vi "Compass.vi"() -> (0 "Error Out":errorcluster)   [LabVIEW 2017]
uses:
  <vilib>/Platform/TimedLoop/XDataNode/timing_clust.ctl
  <vilib>/Platform/TimedLoop/XDataNode/nitl_modes.ctl
  <vilib>/Platform/TimedLoop/XDataNode/wakeup.ctl
  <vilib>/myRIO/Instrument Drivers/Onboard IO/I2C/typedefs/I2C User Configuration.ctl
  <vilib>/myRIO/Instrument Drivers/Onboard IO/I2C/typedefs/I2C Transfer Rate.ctl
  <vilib>/myRIO/Instrument Drivers/Onboard IO/I2C/typedefs/I2C Reference.ctl
  <vilib>/myRIO/Common/Instrument Driver Framework/Utilities/typedefs/myRIO Generic Hardware Reference.ctl
  <vilib>/myRIO/Common/Instrument Driver Framework/Utilities/typedefs/Hardware Version Enum.ctl
  <vilib>/myRIO/Common/Instrument Driver Framework/Utilities/typedefs/myRIO v1.0 Reference.ctl
  <vilib>/myRIO/Common/Instrument Driver Framework/Utilities/typedefs/Generic FPGA Reference.ctl
  <vilib>/myRIO/Common/Instrument Driver Framework/myRIO v1.0/I2C/typedefs/I2C Channels Enum.ctl
  <vilib>/myRIO/Instrument Drivers/Onboard IO/I2C/typedefs/I2C Configuration.ctl
  <vilib>/userdefined/High Color/nirio_resource_hc.ctl
  <vilib>/myRIO/Instrument Drivers/Onboard IO/DIO/typedefs/DIO Reference.ctl
  <vilib>/myRIO/Common/Instrument Driver Framework/myRIO v1.0/DIO/typedefs/DIO Channels List.ctl
  <vilib>/myRIO/Common/Instrument Driver Framework/myRIO v1.0/DIO/typedefs/DIO Channels Enum.ctl
  <vilib>/myRIO/Common/Instrument Driver Framework/Utilities/vis/Is FPGA Ref Available.vi
  <vilib>/myRIO/Common/Instrument Driver Framework/myRIO v1.0/I2C/vis/myRIO v1.1 Open I2C.vi
  <vilib>/myRIO/Instrument Drivers/Onboard IO/I2C/vis/Configure.vi
  <vilib>/myRIO/Instrument Drivers/Onboard IO/I2C/vis/Write.vi
  <vilib>/myRIO/Common/Instrument Driver Framework/myRIO v1.0/DIO/vis/myRIO v1.1 Open DIO.vi
  <vilib>/myRIO/Instrument Drivers/Onboard IO/DIO/vis/Read.vi
  <vilib>/myRIO/Common/Instrument Driver Framework/Utilities/vis/Validate Channels.vi
  <vilib>/myRIO/Common/Instrument Driver Framework/myRIO v1.0/I2C/vis/myRIO v1.0 Reserve I2C.vi
  <vilib>/myRIO/Common/Instrument Driver Framework/myRIO v1.0/DIO/vis/myRIO v1.0 Reserve DIO.vi
  <vilib>/myRIO/Instrument Drivers/Onboard IO/I2C/vis/Write Read.vi
  <vilib>/myRIO/Common/Instrument Driver Framework/myRIO v1.0/I2C/vis/myRIO v1.0 Build MUX Configuration I2C.vi
  <vilib>/myRIO/Common/Instrument Driver Framework/myRIO v1.0/Resource Manager/vis/myRIO v1.0 Reserve Channel List.vi
  <vilib>/myRIO/Common/Instrument Driver Framework/myRIO v1.0/DIO/vis/myRIO v1.0 Build MUX Configuration DIO.vi
  <vilib>/myRIO/Common/Instrument Driver Framework/myRIO v1.0/Resource Manager/vis/myRIO v1.0 Create Configuration List.vi
  <vilib>/myRIO/Common/Instrument Driver Framework/myRIO v1.0/Resource Manager/vis/myRIO v1.0 Reserve Channel.vi
  <vilib>/myRIO/Common/Instrument Driver Framework/myRIO v1.0/Resource Manager/vis/myRIO v1.0 Unreserve Channel.vi
  <vilib>/myRIO/Common/Instrument Driver Framework/myRIO v1.0/Resource Manager/vis/myRIO v1.0 Build Mutex Name.vi
  <vilib>/Utility/VariantDataType/GetNumericInfo.vi
  <vilib>/Utility/error.llb/Error Cluster From Error Code.vi
  <vilib>/myRIO/Common/Instrument Driver Framework/myRIO v1.0/myRIO v1.1 Open.vi
  <vilib>/myRIO/Common/Instrument Driver Framework/Utilities/vis/IO Manager.vi
  <vilib>/myRIO/Common/Instrument Driver Framework/Utilities/vis/Configuration Manager.vi
  <vilib>/myRIO/Common/Instrument Driver Framework/myRIO v1.0/Resource Manager/vis/myRIO v1.0 Configure IO.vi
  <vilib>/myRIO/Common/Instrument Driver Framework/myRIO v1.0/myRIO v1.0 Close.vi
  <vilib>/myRIO/Common/Instrument Driver Framework/myRIO v1.0/I2C/vis/myRIO v1.0 Configure I2C.vi
  <vilib>/myRIO/Common/Instrument Driver Framework/myRIO v1.0/I2C/vis/myRIO v1.0 Write I2C.vi
  <vilib>/myRIO/Common/Instrument Driver Framework/myRIO v1.0/DIO/vis/myRIO v1.0 Read DIO.vi
  <vilib>/myRIO/Instrument Drivers/Onboard IO/I2C/vis/Smart Open.vi
  <vilib>/myRIO/Common/Instrument Driver Framework/myRIO v1.0/I2C/vis/myRIO v1.0 Read I2C.vi
  <vilib>/Platform/TimedLoop/XDataNode/XDataNode.xnode
  <vilib>/myRIO/Express VI/Onboard IO/I2C/I2C Express VI.xnode
  <vilib>/myRIO/Instrument Drivers/Onboard IO/I2C/vis/myRIO I2C Open.xnode
  <vilib>/myRIO/Express VI/Onboard IO/DI/DI Express VI.xnode
  <vilib>/myRIO/Instrument Drivers/Onboard IO/DIO/vis/myRIO DIO Open.xnode
  <vilib>/Platform/TimedLoop/XDataNode/XDNodeRunTimeDep.lvlib
  <vilib>/myRIO/Instrument Drivers/Onboard IO/I2C/I2C.lvlib
  <vilib>/myRIO/Instrument Drivers/Onboard IO/DIO/DIO.lvlib
panel:
  out "Angle (deg) without declination added":dbl
  out "Angle + 90 (deg)":dbl
  out "Angle (deg)":dbl
  out "atan2(y,x)":dbl
  out "cali_Y":dbl
  out "cali_X":dbl
  out "avg(Y)":dbl
  out "avg(X)":dbl
  out "max(Y)":i16
  out "min(Y)":i16
  out "min(X)":i16
  out "max(X)":i16
  out "Magnetic field [LSb]":cluster{i16, i16, i16}(graph) caption="Waveform Chart"
  out "Z":i16
  out "Y":i16
  out "X":i16
  out "DATA":u8[](array[numeric]) format="%02x"
  # "Compass demo"
  # "DATA_X_H"
  # "DATA_X_L"
  # "DATA_Z_H"
  # "DATA_Z_L"
  # "DATA_Y_H"
  # "DATA_Y_L"
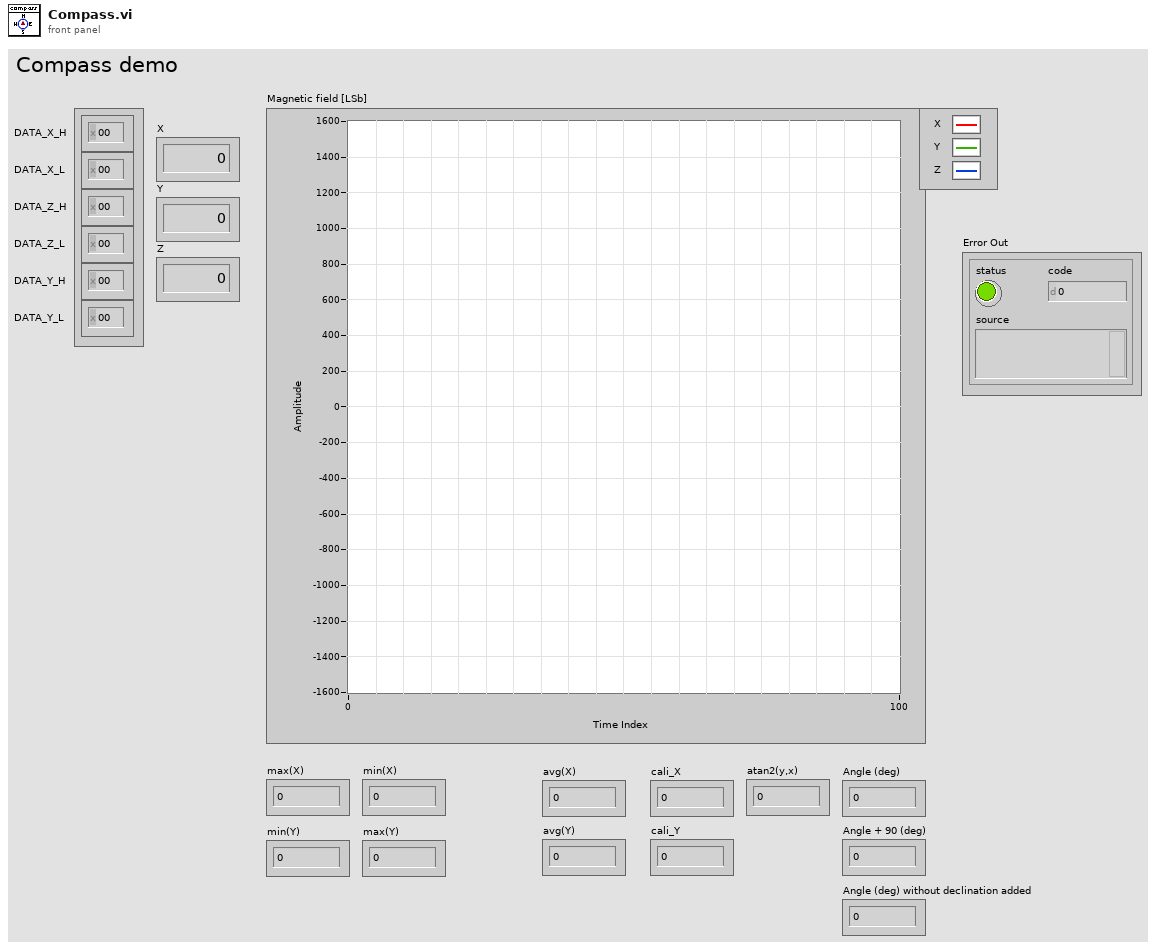
[diagram p1: front panel]
types:
  T1 = typedef "XDNodeRunTimeDep.lvlib/timing_clust.ctl" = cluster{"Expected End [f-1]":u64, "Actual End [f-1]":u64, "Finished Late? [f-1]":bool, "Expected End [i-1]":u64, "Actual End [i-1]":u64, "Finished Late? [i-1]":bool, "Expected Start [i]":u64, "Actual Start [i]":u64, "Expected Start [f]":u64, "Actual Start [f]":u64, "Source Name":string, "Structure Name":string, "Period":i64, "Deadline":i64, "Offset":i64, "Start":i64, "Priority":i32, "Timeout":i32, "Mode":T2, "Wakeup Reason":T3, "Error":errorcluster, "Source Type":string, "Secondary Source Type":string, "Global End Time":u64, "Global Start Time":u64, "Frame Duration":u64, "Iteration Duration":u64, "Assigned CPU":i32, "I/O Scan Engine Mode":u32}
  T2 = typedef "XDNodeRunTimeDep.lvlib/nitl_modes.ctl" = enum32{"No Change", "Process missed periods, maintain original phase", "Discard missed periods, maintain original phase", "Process missed periods, ignore original phase", "Discard missed periods, ignore original phase"}
  T3 = typedef "XDNodeRunTimeDep.lvlib/wakeup.ctl" = enum32{"Normal", "Aborted", "Asynchronous wakeup", "Timing source error", "Timed loop error", "Timeout"}
  T4 = typedef "DIO.lvlib/DIO Reference.ctl" = cluster{"myRIO Reference":T5, "DIO Channels List":T9}
  T5 = typedef "myRIO Generic Hardware Reference.ctl" = cluster{"myRIO Model":T6, "myRIO Hardware Reference":T7}
  T6 = typedef "Hardware Version Enum.ctl" = enum16{"Unknown", "myRIO-1900", "myRIO-1950", "roboRIO", "NI ELVIS RIO CM"}
  T7 = typedef "myRIO v1.0 Reference.ctl" = cluster{"Generic FPGA Reference":T8, "Allow multiple opens":bool}
  T8 = typedef "Generic FPGA Reference.ctl" = refnum<k20>
  T9 = typedef "DIO Channels List.ctl" = T10[]
  T10 = typedef "DIO Channels Enum.ctl" = enum16{"Not Connected", "C/DIO0", "C/DIO1", "C/DIO2", "C/DIO3", "C/DIO4", "C/DIO5", "C/DIO6", "C/DIO7", "A/DIO0", "A/DIO1", "A/DIO2", "A/DIO3", "A/DIO4", "A/DIO5", "A/DIO6", "A/DIO7", "A/DIO8", "A/DIO9", "A/DIO10", "A/DIO11", "A/DIO12", "A/DIO13", "A/DIO14", "A/DIO15", "B/DIO0", "B/DIO1", "B/DIO2", "B/DIO3", "B/DIO4", "B/DIO5", "B/DIO6", "B/DIO7", "B/DIO8", "B/DIO9", "B/DIO10", "B/DIO11", "B/DIO12", "B/DIO13", "B/DIO14", "B/DIO15", "LED0", "LED1", "LED2", "LED3", "Button0", "DIO/DIO0", "DIO/DIO1", "DIO/DIO2", "DIO/DIO3", "DIO/DIO4", "DIO/DIO5", "DIO/DIO6", "DIO/DIO7", "DIO/DIO8", "DIO/DIO9", "SPI/CS0", "SPI/CS1", "SPI/CS2", "SPI/CS3", "LED RADIO (Green)", "LED RADIO (Red)", "LED COMM (Green)", "LED COMM (Red)", "LED MODE (Green)", "LED MODE (Red)"}
  T11 = typedef "nirio_resource_hc.ctl" = tag
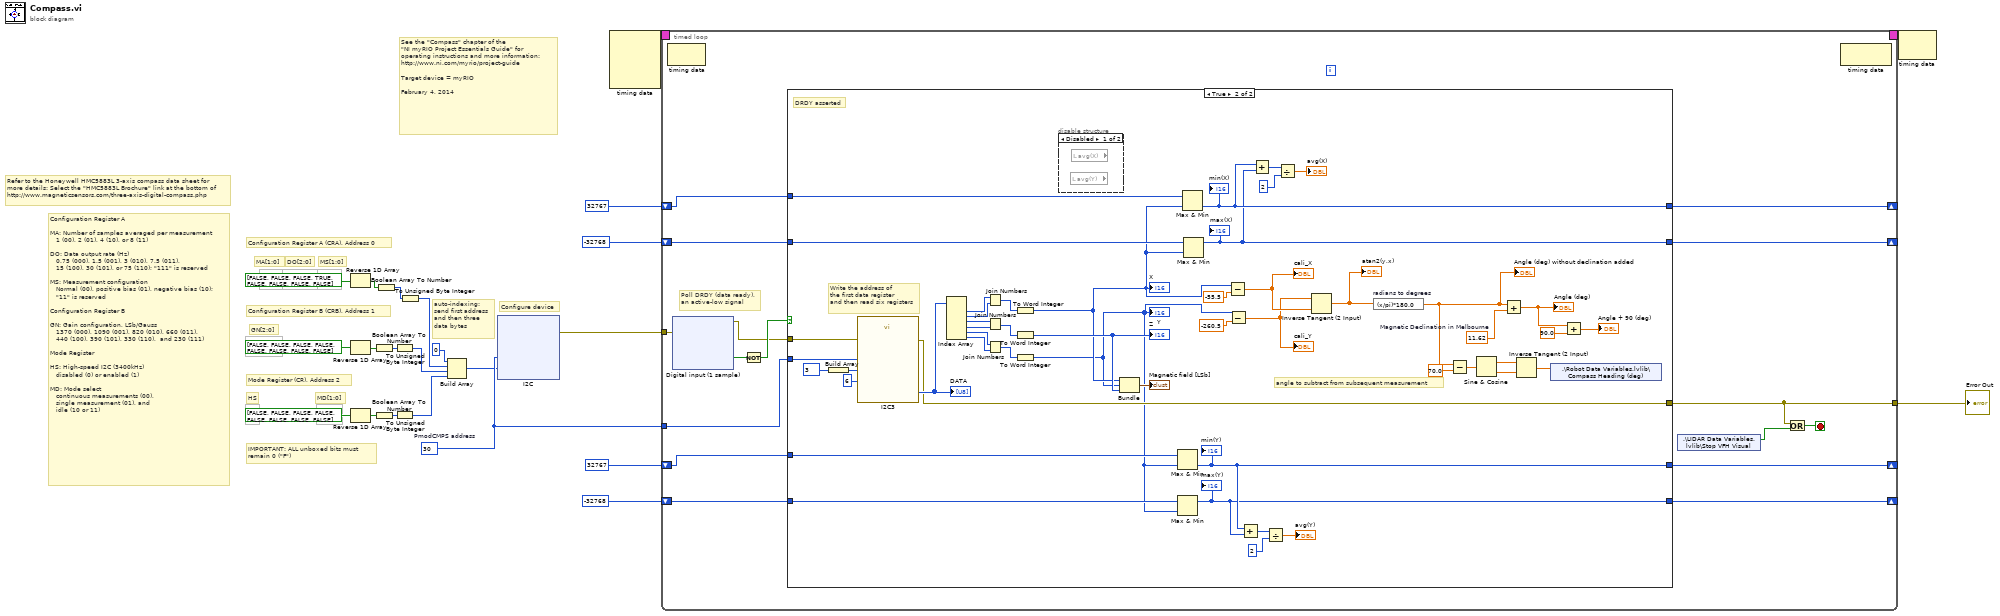
[diagram p0: block diagram]
diagram:
  w22 = u8 30  # PmodCMPS address
  # "See the \"Compass\" chapter of the\n\"NI myRIO Project Essentials Guide\" for\noperating instructions and more information: \nhttp://www.ni.com/myrio/project-guide\n\nTarget device = myRIO\n\nFebruary 4, 2014"
  # "Refer to the Honeywell HMC5883L 3-axis compass data sheet for \nmore details: Select the \"HMC5883L Brochure\" link at the bottom of\nhttp://www.magneticsensors.com/three-axis-digital-compass.php"
  # "auto-indexing:\nsend first address\nand then three\ndata bytes"
  # "Configuration Register A\n\nMA: Number of samples averaged per measurement\n   1 (00), 2 (01), 4 (10), or 8 (11)\n\nDO: Data output rate (Hz)\n   0.75 (000), 1.5 (001), 3 (010), 7.5 (011),\n   15 (100), 30 (101), or 75 (110); \"111\" is reserved\n\nMS: Measurement configuration\n   Normal (00), positive bias (01), negative bias (10);\n   \"11\" is reserved\n\nConfiguration Register B\n\nGN: Gain configuration, LSb/Gauss\n   1370 (000), 1090 (001), 820 (010), 660 (011),\n   440 (100), 390 (101), 330 (110),  and 230 (111)\n\nMode Register\n\nHS: High-speed I2C (3400kHz)\n   disabled (0) or enabled (1)\n\nMD: Mode select\n   continuous measurements (00),\n   single measurement (01), and\n   idle (10 or 11)"
  # "IMPORTANT: ALL unboxed bits must\nremain 0 (\"F\")"
  # "Configure device"
  # "MD[1:0]"
  # "Mode Register (CR), Address 2"
  # "HS"
  # "Configuration Register B (CRB), Address 1"
  # "GN[2:0]"
  # "Configuration Register A (CRA), Address 0"
  # "MS[1:0]"
  # "DO[2:0]"
  # "MA[1:0]"
  n1 = Reverse 1D Array(array=bool[] [FALSE, FALSE, FALSE, TRUE, FALSE, FALSE, FALSE, FALSE]) -> (reversed array=w17:bool[])
  n2 = Reverse 1D Array(array=bool[] [FALSE, FALSE, FALSE, FALSE, FALSE, FALSE, FALSE, FALSE]) -> (reversed array=w16:bool[])
  n3 = Reverse 1D Array(array=bool[] [FALSE, FALSE, FALSE, FALSE, FALSE, FALSE, FALSE, FALSE]) -> (reversed array=w14:bool[])
  n4 = Boolean Array To Number(Boolean array=w16) -> (number=w10:u32)
  n5 = Boolean Array To Number(Boolean array=w14) -> (number=w9:u32)
  n6 = Boolean Array To Number(Boolean array=w17) -> (number=w11:u32)
  n7 = To Unsigned Byte Integer(number=w10) -> (unsigned 8bit integer=w7:u8)
  n8 = To Unsigned Byte Integer(number=w9) -> (unsigned 8bit integer=w6:u8)
  n9 = To Unsigned Byte Integer(number=w11) -> (unsigned 8bit integer=w8:u8)
  n10 = Build Array "Build Array"(u8 0 ("address"), w8, w7, w6) -> (w21:u8[])
  n11 = xnode "I2C"("Slave Address (7-bit)"=w22, "Bytes to Write"=w21) -> ("error out"=w23:errorcluster)  [unwired: 1 in]
  n12 = node-c288() -> (w20:T1)  [unwired: 4 in]
  n13 = timed-loop {
    tunnel: [w33] -> w1
    tunnel: w23 -> [w37]
    tunnel: w22 -> [w38]
    timing: w20 -> [_]
    timing-out: [_] -> w19
    shift-right: [w32] -> _
    shift-left: i16 -32768 -> [w31]
    shift-right: [w30] -> _
    shift-left: i16 32767 -> [w29]
    shift-right: [w27] -> _
    shift-left: i16 32767 -> [w26]
    shift-right: [w28] -> _
    shift-left: i16 -32768 -> [w25]
    stop <- w39 stop-if-true
    # "Poll DRDY (data ready),\nan active-low signal"
    n14 = node-c288() -> ()  [unwired: 1 in, 1 out]
    n15 = xnode "Digital input (1 sample)"("error in (no error)"=w37) -> ("A/DIO7 (Pin 25)"=w36:bool, "error out"=w34:errorcluster)
    n16 = Not(x=w36) -> (.not. x?=w35:bool)
    n17 = case shown="True" w35 {
      tunnel: w38 -> [_ w130]
      tunnel: w34 -> [w81 w119]
      tunnel: [w81 w115] -> w33
      tunnel: [w80 w106] -> w32
      tunnel: w31 -> [w80 w113]
      tunnel: [w79 w107] -> w30
      tunnel: w29 -> [w79 w111]
      tunnel: [w77 w100] -> w28
      tunnel: [w78 w101] -> w27
      tunnel: w26 -> [w78 w110]
      tunnel: w25 -> [w77 w109]
      frame False {
        # "DRDY deasserted"
      }
      frame True {
        w93 = 11.62  # Magnetic Declination in Melbourne
        # "angle to subtract from subsequent measurement"
        # "DRDY asserted"
        # "Write the address of\nthe first data register\nand then read six registers"
        n18 = Build Array(u8 3) -> (w116:u8[])
        n19 = call "I2C3"("Slave Address (7-bit)"=w130, "Bytes to Write"=w116, "Byte Count"=u32 6, "error in (no error)"=w119) -> ("Bytes Read"=w120:u8[], "error out"=w115:errorcluster)  [unwired: 22 in]
        "DATA" <- w120
        n20 = Index Array "Index Array"(array=w120) -> (element #1=w129:u8, element #2=w128:u8, element #3=w126:u8, element #4=w125:u8, element #5=w124:u8, element #6=w123:u8)  [unwired: 6 in]
        n21 = Join Numbers(hi=w129, lo=w128) -> ((hi.lo)=w127:u16)
        n22 = Join Numbers(hi=w126, lo=w125) -> ((hi.lo)=w122:u16)
        n23 = Join Numbers(hi=w124, lo=w123) -> ((hi.lo)=w121:u16)
        n24 = To Word Integer(number=w127) -> (16bit integer=w98:i16)
        "X" <- w98
        n25 = To Word Integer(number=w122) -> (16bit integer=w112:i16)
        "Z" <- w112
        n26 = To Word Integer(number=w121) -> (16bit integer=w97:i16)
        "Y" <- w97
        n27 = disable-structure shown="Disabled" {
          frame Disabled {
            n28 = local read "avg(Y)"() -> ()  [unwired: 1 out]
            n29 = local read "avg(X)"() -> ()  [unwired: 1 out]
          }
          frame Enabled {
          }
        }
        n30 = Bundle(w98, w97, w112) -> (→"Magnetic field [LSb]":cluster{i16, i16, i16})  [unwired: 1 in]
        n31 = Max & Min(x=w110, y=w97) -> (min(x,y)=w101:i16)  [unwired: 1 out]
        "min(Y)" <- w101
        n32 = Max & Min(x=w109, y=w97) -> (max(x,y)=w100:i16)  [unwired: 1 out]
        "max(Y)" <- w100
        n33 = Max & Min(x=w111, y=w98) -> (min(x,y)=w107:i16)  [unwired: 1 out]
        "min(X)" <- w107
        n34 = Max & Min(x=w113, y=w98) -> (max(x,y)=w106:i16)  [unwired: 1 out]
        "max(X)" <- w106
        n35 = Subtract(x=w98, y=-55.5 ("Magnetic Declination in Melbourne")) -> (x-y=w95:dbl)
        "cali_X" <- w95
        n36 = Subtract(x=w97, y=-260.5 ("Magnetic Declination in Melbourne")) -> (x-y=w94:dbl)
        "cali_Y" <- w94
        n37 = Add(x=w101, y=w100) -> (x+y=w103:i16)
        n38 = Add(x=w107, y=w106) -> (x+y=w108:i16)
        n39 = Divide(x=w103, y=i16 2) -> (x/y=→"avg(Y)":dbl)
        n40 = Divide(x=w108, y=i16 2) -> (x/y=→"avg(X)":dbl)
        n41 = Inverse Tangent (2 Input)(1:w95, 2:w94) -> (0:w96:dbl)
        "atan2(y,x)" <- w96
        n42 = expression code="(x/pi)*180.0" "radians to degrees"(w96) -> (w87:dbl)
        "Angle (deg) without declination added" <- w87
        n43 = Subtract(x=w87, y=70.0) -> (x-y=w83:dbl)
        n44 = Sine & Cosine(0:w83) -> (1:w85:dbl, 2:w84:dbl)
        n45 = Add(x=w87, y=w93) -> (x+y=w92:dbl)
        "Angle (deg)" <- w92
        n46 = Inverse Tangent (2 Input)(1:w84, 2:w85) -> (0:w82:dbl)
        n47 = shared-variable ".\\Robot Data Variables.lvlib\\Compass Heading (deg)"(w82) -> ()  [unwired: 1 in, 1 out]
        n48 = Add(x=w92, y=90.0) -> (x+y=→"Angle + 90 (deg)":dbl)
      }
    }
    n49 = shared-variable ".\\LIDAR Data Variables.lvlib\\Stop VFH Visual"() -> (w24:bool)  [unwired: 1 in, 1 out]
    n50 = Or(x=w33, y=w24) -> (x .or. y?=w39:bool)
    n51 = node-c288() -> ()  [unwired: 1 in, 1 out]
  }
  "Error Out" <- w1
  n52 = node-c288(w19) -> ()  [unwired: 1 out]
